vi "rs3 Advanced get Color control3.vi"(8 "error in (no error)":errorcluster, 10 "mode":i32, 11 "device in":u64) -> (0 "error out 2":errorcluster, 1 "error":u64, 2 "ST Color Control":T1, 3 "Dev out":u64)   [LabVIEW 2017, in "libRealSense3.lvlib"]
doc: "Opens communication to a specific RealSense Device."
uses:
  libRealSense3.lvlib
  realsense2.dll
panel:
  # "RS3 Adv. Get Color Control 2"
  # "(C) 2017 Intel Corp.,  AGJ"
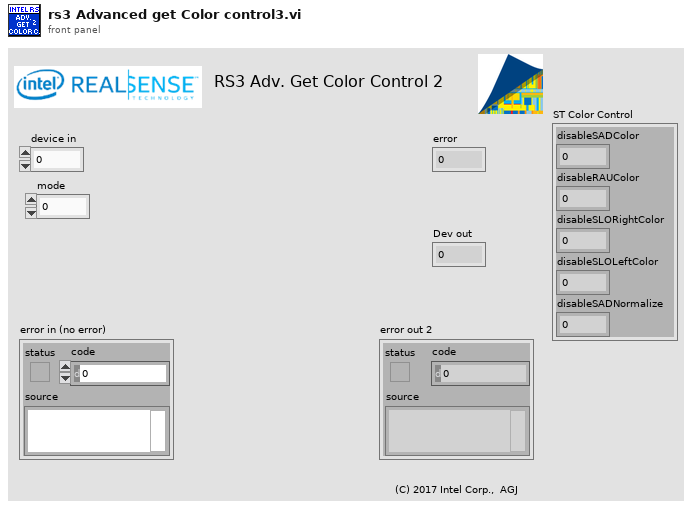
[diagram p1: front panel]
types:
  T1 = cluster{"disableSADColor":u32, "disableRAUColor":u32, "disableSLORightColor":u32, "disableSLOLeftColor":u32, "disableSADNormalize":u32}
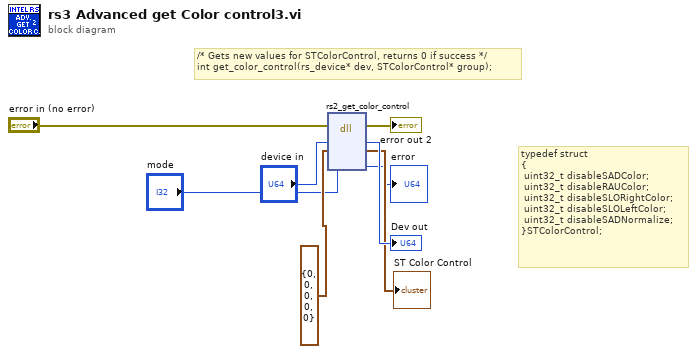
[diagram p0: block diagram]
diagram:
  # "typedef struct\n{\n\tuint32_t disableSADColor;\n\tuint32_t disableRAUColor;\n\tuint32_t disableSLORightColor;\n\tuint32_t disableSLOLeftColor;\n\tuint32_t disableSADNormalize;\n}STColorControl;"
  # "/* Gets new values for STColorControl, returns 0 if success */\nint get_color_control(rs_device* dev, STColorControl* group);"
  n1 = dll-call lib="C:/Users/agrunnet/Documents/libRealSense6/realsense2.dll" fn="rs2_get_color_control"(error in="error in (no error)", "device"="device in", "ST Color Control"=T1 {"disableSADColor"=0, "disableRAUColor"=0, "disableSLORightColor"=0, "disableSLOLeftColor"=0, "disableSADNormalize"=0} ("output cluster"), "mode"="mode") -> (error out=→"error out 2":errorcluster, "device"=→"Dev out":u64, "ST Color Control"=→"ST Color Control":T1, "error"=→"error":u64)  [unwired: 5 in, 1 out]
